vi "parseFloat.vi"(8 "error in (no error)":errorcluster, 9 "unit":T1, 10 "commandData":string, 11 "CoolerSerialCommand in":refnum<class "CoolerSerialCommand.lvclass">) -> (0 "error out":errorcluster, 1 "statusActive":bool, 2 "value":sgl, 3 "CoolerSerialCommand out":refnum<class "CoolerSerialCommand.lvclass">)   [LabVIEW 2016, in "CoolerSerialCommand.lvclass"]
uses:
  CoolerSerialCommand.lvclass
  typedefs/dataUnit.ctl
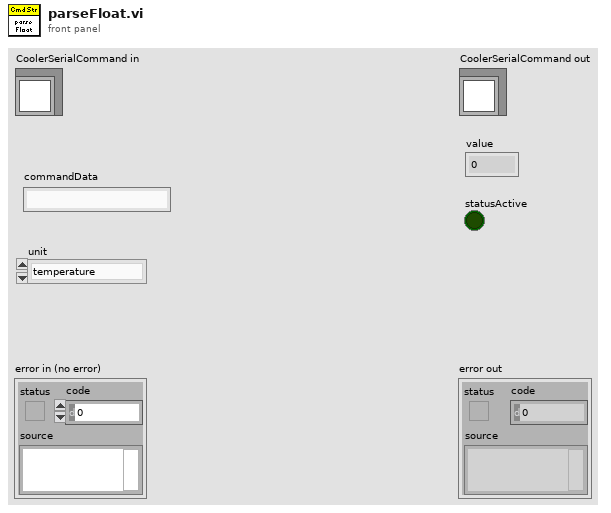
[diagram p1: front panel]
types:
  T1 = typedef "dataUnit.ctl" = enum16{"temperature", "flow", "current", "PID", "fanSpeed", "time", "PWM", "TEDriveLevel", "Number"}
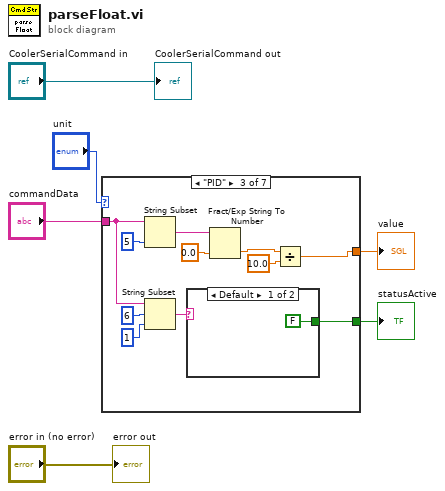
[diagram p0: block diagram]
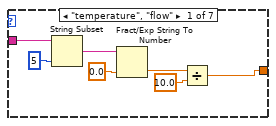
[diagram p2: hidden frame]
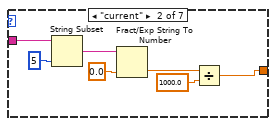
[diagram p3: hidden frame]
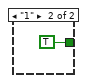
[diagram p4: hidden frame]
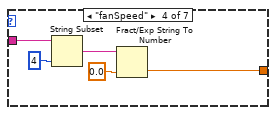
[diagram p5: hidden frame]
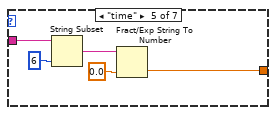
[diagram p6: hidden frame]
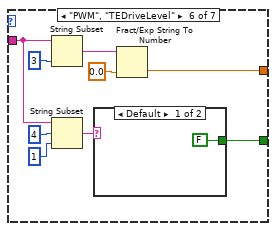
[diagram p7: hidden frame]
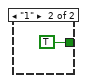
[diagram p8: hidden frame]
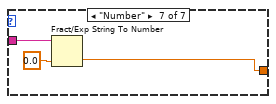
[diagram p9: hidden frame]
diagram:
  n1 = case shown="\"PID\"" "unit" {
    tunnel: "commandData" -> [w12 w15 w24 w35 w40 w47 w56]
    tunnel: [w8 w14 w26 w34 w39 w49 w55] -> w3
    tunnel: [_ _ w21 _ _ w44 _] -> w1
    frame "temperature", "flow" {
      n2 = String Subset(string=w12, length (rest)=5 ("length (rest)")) -> (substring=w10:string)  [unwired: 1 in]
      n3 = Fract/Exp String To Number(string=w10, default (0 dbl)=sgl 0.0 ("value")) -> (number=w9:sgl)  [unwired: 2 in, 1 out]
      n4 = Divide(x=w9, y=sgl 10.0) -> (x/y=w8:sgl)
    }
    frame "current" {
      n5 = String Subset(string=w15, length (rest)=5 ("length (rest)")) -> (substring=w18:string)  [unwired: 1 in]
      n6 = Fract/Exp String To Number(string=w18, default (0 dbl)=sgl 0.0 ("value")) -> (number=w17:sgl)  [unwired: 2 in, 1 out]
      n7 = Divide(x=w17, y=sgl 1000.0) -> (x/y=w14:sgl)
    }
    frame "PID" {
      n8 = String Subset(string=w24, length (rest)=5 ("length (rest)")) -> (substring=w29:string)  [unwired: 1 in]
      n9 = String Subset(string=w24, offset (0)=6, length (rest)=1 ("length (rest)")) -> (substring=w22:string)
      n10 = case shown="Default" w22 {
        tunnel: [FALSE TRUE] -> w21
        frame Default {
        }
        frame "1" {
        }
      }
      n11 = Fract/Exp String To Number(string=w29, default (0 dbl)=sgl 0.0 ("value")) -> (number=w28:sgl)  [unwired: 2 in, 1 out]
      n12 = Divide(x=w28, y=sgl 10.0) -> (x/y=w26:sgl)
    }
    frame "fanSpeed" {
      n13 = String Subset(string=w35, length (rest)=4 ("length (rest)")) -> (substring=w36:string)  [unwired: 1 in]
      n14 = Fract/Exp String To Number(string=w36, default (0 dbl)=sgl 0.0 ("value")) -> (number=w34:sgl)  [unwired: 2 in, 1 out]
    }
    frame "time" {
      n15 = String Subset(string=w40, length (rest)=6 ("length (rest)")) -> (substring=w41:string)  [unwired: 1 in]
      n16 = Fract/Exp String To Number(string=w41, default (0 dbl)=sgl 0.0 ("value")) -> (number=w39:sgl)  [unwired: 2 in, 1 out]
    }
    frame "PWM", "TEDriveLevel" {
      n17 = String Subset(string=w47, length (rest)=3 ("length (rest)")) -> (substring=w52:string)  [unwired: 1 in]
      n18 = String Subset(string=w47, offset (0)=4, length (rest)=1 ("length (rest)")) -> (substring=w45:string)
      n19 = case shown="Default" w45 {
        tunnel: [FALSE TRUE] -> w44
        frame Default {
        }
        frame "1" {
        }
      }
      n20 = Fract/Exp String To Number(string=w52, default (0 dbl)=sgl 0.0 ("value")) -> (number=w49:sgl)  [unwired: 2 in, 1 out]
    }
    frame "Number" {
      n21 = Fract/Exp String To Number(string=w56, default (0 dbl)=sgl 0.0 ("value")) -> (number=w55:sgl)  [unwired: 2 in, 1 out]
    }
  }
  "value" <- w3
  "statusActive" <- w1
  "error out" <- "error in (no error)"
  "CoolerSerialCommand out" <- "CoolerSerialCommand in"
